vi "Update Height by Slider.vi"(4 "Bottom Numeric":sgl, 5 "Logarithm?":bool, 6 "Top Numeric":sgl=100.0, 7 "Slider Ref":refnum<vi>, 8 "error in (no error)":errorcluster, 9 "Numeric Ref Array":refnum<vi>[](array[refnum]), 10 "Color Ref Array":refnum<vi>[](array[refnum]), 11 "Slider Ref Array":refnum<vi>[](array[refnum])) -> (0 "error out":errorcluster)   [LabVIEW 2017, in "3D Plot.lvclass"]
uses:
  <vilib>/Math Plots/3D Math Plots/3D Plot/3D Plot/3D Plot.lvclass
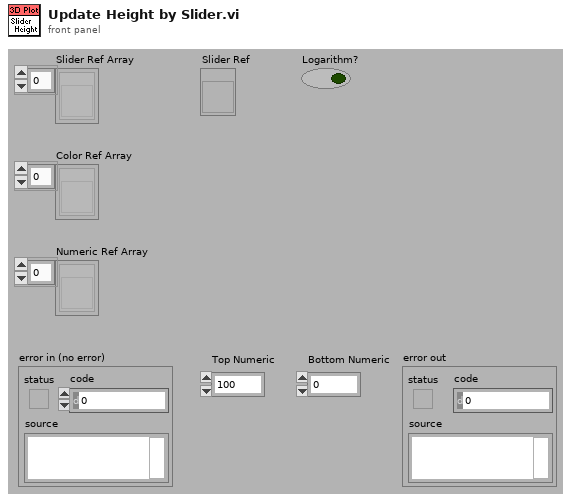
[diagram p1: front panel]
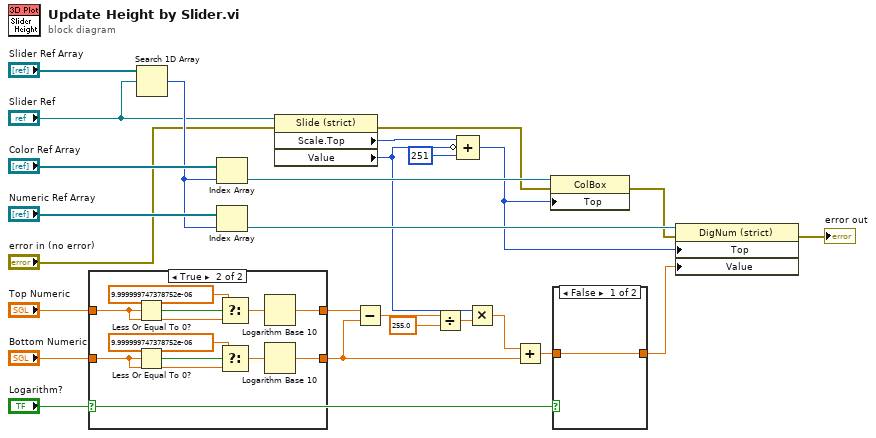
[diagram p0: block diagram]
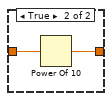
[diagram p2: hidden frame]
diagram:
  n1 = case shown="True" "Logarithm?" {
    tunnel: "Top Numeric" -> [w28 w29]
    tunnel: [w28 w38] -> w6
    tunnel: "Bottom Numeric" -> [w27 w30]
    tunnel: [w27 w37] -> w4
    frame False {
    }
    frame True {
      n2 = Less Or Equal To 0?(x=w29) -> (x <= 0?=w33:bool)
      n3 = Less Or Equal To 0?(x=w30) -> (x <= 0?=w36:bool)
      n4 = Select(t=sgl 1e-05, s=w33, f=w29) -> (s? t:f=w32:sgl)
      n5 = Select(t=sgl 1e-05, s=w36, f=w30) -> (s? t:f=w31:sgl)
      n6 = Logarithm Base 10(1:w32) -> (0:w38:sgl)
      n7 = Logarithm Base 10(1:w31) -> (0:w37:sgl)
    }
  }
  n8 = Search 1D Array(1D array="Slider Ref Array", element="Slider Ref") -> (index of element=w23:i32)  [unwired: 1 out]
  n9 = Index Array(array="Color Ref Array", index=w23) -> (element=w22:refnum<vi>)
  n10 = Index Array(array="Numeric Ref Array", index=w23) -> (element=w21:refnum<vi>)
  n11 = property class="Slide (strict)"(reference="Slider Ref", error in="error in (no error)") -> (error out=w16:errorcluster, "Scale.Top"=w19:i32, "Value"=w9:i32)  [unwired: 1 out]
  n12 = Subtract(x=w6, y=w4) -> (x-y=w12:sgl)
  n13 = Divide(x=w12, y=sgl 255.0) -> (x/y=w10:sgl)
  n14 = Compound Arithmetic op=ADD(w19, invert w9, 251 ("value")) -> (w18:i32)
  n15 = Multiply(x=w9, y=w10) -> (x*y=w8:sgl)
  n16 = Add(x=w8, y=w4) -> (x+y=w2:sgl)
  n17 = property class="ColBox"(reference=w22, error in=w16, "Top"=w18) -> (error out=w15:errorcluster)  [unwired: 1 out]
  n18 = case shown="False" "Logarithm?" {
    tunnel: w2 -> [w39 w41]
    tunnel: [w39 w40] -> w1
    frame False {
    }
    frame True {
      n19 = Power Of 10(x=w41) -> (10^x=w40:sgl)
    }
  }
  n20 = property class="DigNum (strict)"(reference=w21, error in=w15, "Top"=w18, "Value"=w1) -> (error out=→"error out":errorcluster)  [unwired: 1 out]
